vi "SingleOutPut.vi"(8 "error in (no error)":errorcluster, 9 "Bool":bool, 10 "Index":i32, 11 "ZanCard in":refnum<class "ZanCard.lvclass">) -> (0 "error out":errorcluster, 3 "ZanCard out":refnum<class "ZanCard.lvclass">)   [LabVIEW 2019, in "ZanCard.lvclass"]
uses:
  ZanCard.lvclass
  ZanCard.lvclass/ZanCard.ctl
  LLB/zmotion/zaux/zauxdll.lvlib
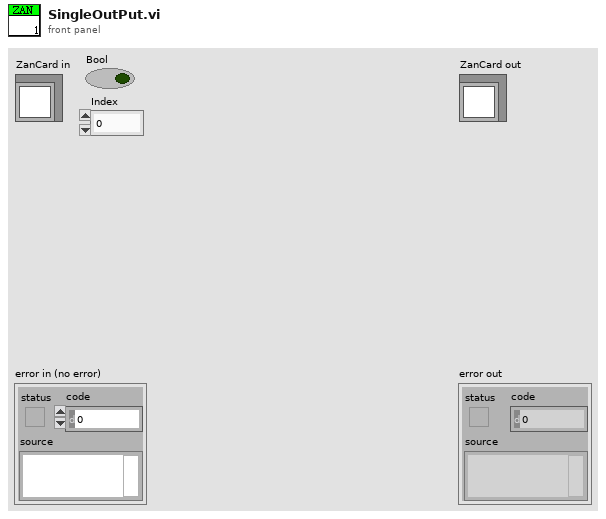
[diagram p1: front panel]
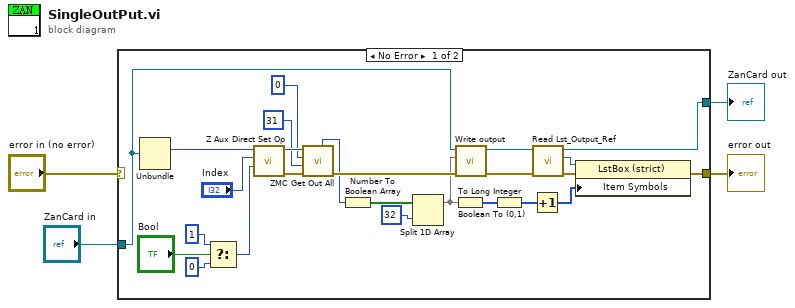
[diagram p0: block diagram]
diagram:
  n1 = case shown="No Error" "error in (no error)" {
    selector: "error in (no error)" -> [_ w31]
    tunnel: "ZanCard in" -> [w25 w30]
    tunnel: [w22 w30] -> w2
    tunnel: [w19 w31] -> w1
    frame No Error {
      n2 = Unbundle(w25) -> (w29:i32)  [unwired: 3 out]
      n3 = Select(t=1, s="Bool", f=0) -> (s? t:f=w26:i32)
      n4 = call "Z Aux Direct Set Op.vi"("iValue"=w26, "ionum"="Index", "handle"=w29) -> ("error out"=w12:errorcluster, "handle out"=w18:u32)  [unwired: 6 in, 1 out]
      n5 = call "ZMC Get Out All.vi"("error in (no error)"=w12, "inumend"=31 ("ionumend"), "inumfirst"=0 ("ionumfirst"), "handle"=w18) -> ("error out"=w13:errorcluster, "pistate out"=w11:u32)  [unwired: 4 in, 2 out]
      n6 = Number To Boolean Array(number=w11) -> (Boolean array=w15:bool[])
      n7 = Split 1D Array(array=w15, index=32) -> (first subarray=w6:bool[])  [unwired: 1 out]
      n8 = Boolean To (0,1)(Boolean=w6) -> (0, 1=w8:i16[])
      n9 = call-dynamic "Write output.vi"("error in (no error)"=w13, "output"=w6, "IOCard in"=w25) -> ("error out"=w21:errorcluster, "IOCard out"=w24:refnum<class "ZanCard.lvclass">)  [unwired: 7 in]
      n10 = To Long Integer(number=w8) -> (32bit integer=w7:i32[])
      n11 = Increment(x=w7) -> (x+1=w5:i32[])
      n12 = call-dynamic "Read Lst_Output_Ref.vi"("error in (no error)"=w21, "IOCard in"=w24) -> ("error out"=w20:errorcluster, "Lst_Output_Ref"=w23:refnum<vi>, "IOCard out"=w22:refnum<class "ZanCard.lvclass">)  [unwired: 7 in]
      n13 = property class="LstBox (strict)"(reference=w23, error in=w20, "Item Symbols"=w5) -> (error out=w19:errorcluster)  [unwired: 1 out]
    }
    frame Error {
    }
  }
  "error out" <- w1
  "ZanCard out" <- w2
